vi "MeasuringDevice.Init.vi"(8 "error in (no error)":errorcluster, 11 "LIA.SR810":refnum<class "LIA.SR810.lvclass">) -> (0 "error out":errorcluster, 3 "LIA.SR810 out":refnum<class "LIA.SR810.lvclass">)   [LabVIEW 2017, in "LIA.SR810.lvclass"]
doc: "---------------------------------------------------------------\nJKI State Machine Objects™\nhttp://jki.net/state-machine-objects/\nCopyright (C) 2005-2015, JKI <info@jki.net>\nALL RIGHTS RESERVEDJKI State Machine Objects (SMO) 1.0.0.5\nJKI - JKI\nCopyright (c) 2016, JKI"
uses:
  LIA.SR810.lvclass
  D:/upwork/Laser Measurement Tool/Laser/project/Subsystems/LIA/LIA.lvclass
  Typedefs/Resource--Cluster.ctl
  LIA/LIA.lvclass
  <instrlib>/Stanford Research 830/Stanford Research 830.lvlib
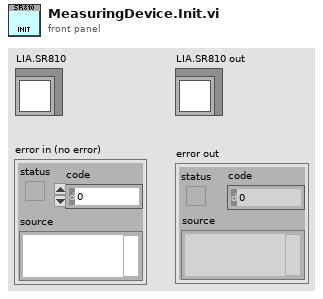
[diagram p1: front panel]
types:
  T1 = typedef "LIA.SR810.lvclass/Resource--Cluster.ctl" = cluster{"VISA resource":refnum<visa-resource-name>}
  T2 = typedef "LIA.lvclass/Configuration--Cluster.ctl" = cluster{"VISA Resource":string}
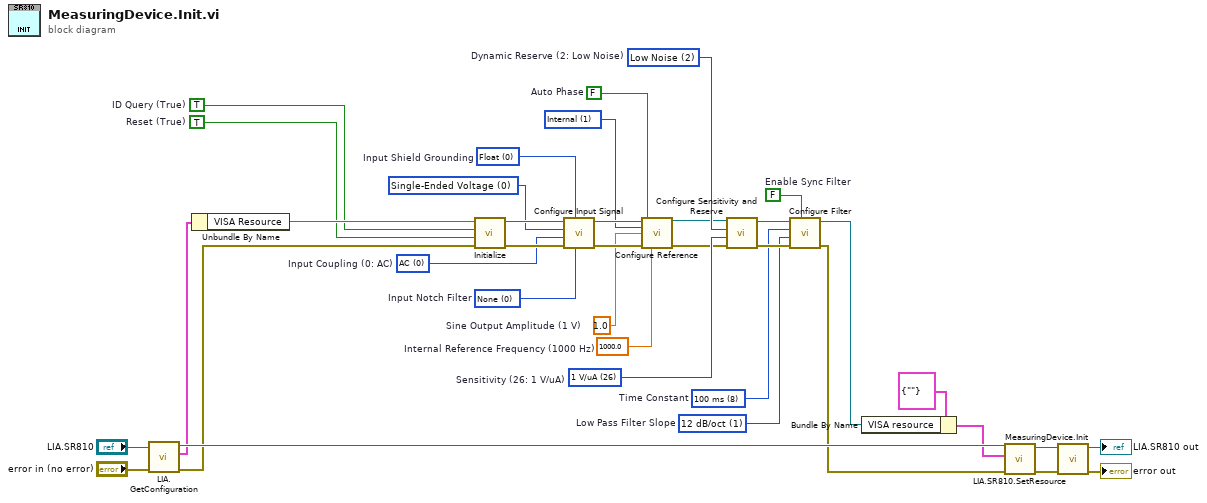
[diagram p0: block diagram]
diagram:
  w1 = TRUE  # Reset (True)
  w2 = TRUE  # ID Query (True)
  w20 = i8 26 items=["Auto Gain"=-1, "2 nV/fA"=0, "5 nV/fA"=1, "10 nV/fA"=2, "20 nV/fA"=3, "50 nV/fA"=4, "100 nV/fA"=5, "200 nV/fA"=6, "500 nV/fA"=7, "1 uV/pA"=8, "2 uV/pA"=9, "5 uV/pA"=10, "10 uV/pA"=11, "20 uV/pA"=12, "50 uV/pA"=13, "100 uV/pA"=14, "200 uV/pA"=15, "500 uV/pA"=16, "1 mV/nA"=17, "2 mV/nA"=18, "5 mV/nA"=19, "10 mV/nA"=20, "20 mV/nA"=21, "50 mV/nA"=22, "100 mV/nA"=23, "200 mV/nA"=24, "500 mV/mA"=25, "1 V/uA"=26]  # Sensitivity (26: 1 V/uA)
  w14 = 1000.0  # Internal Reference Frequency (1000 Hz)
  w15 = 1.0  # Sine Output Amplitude (1 V)
  w24 = u16 0 items=["AC", "DC"]  # Input Coupling (0: AC)
  w25 = u16 0 items=["Single-Ended Voltage", "Differential Voltage", "1 MOhm Current Gain", "100 MOhm Current Gain"] ("Input Connection (0: Single-Ended Voltage)")
  w16 = u16 1 items=["External", "Internal"] ("Reference Source (1: Internal)")
  w19 = i8 2 items=["High Reserve"=0, "Normal"=1, "Low Noise"=2, "Auto Reserve"=-1]  # Dynamic Reserve (2: Low Noise)
  w9 = u16 1 items=["6 dB/oct", "12 dB/oct", "18 db/oct", "24 dB/oct"]  # Low Pass Filter Slope
  w10 = u16 8 items=["10 us", "30 us", "100 us", "300 us", "1 ms", "3 ms", "10 ms", "30 ms", "100 ms", "300 ms", "1 s", "3 s", "10 s", "30 s", "100 s", "300 s", "1 ks", "3 ks", "10 ks", "30 ks"]  # Time Constant
  w11 = FALSE  # Enable Sync Filter
  w21 = FALSE  # Auto Phase
  w22 = u16 0 items=["None", "Line Notch", "2x Line Notch", "Both Notch Filters"]  # Input Notch Filter
  w23 = u16 0 items=["Float", "Ground"]  # Input Shield Grounding
  n1 = call "LIA.GetConfiguration.vi"("error in (no error)"="error in (no error)", "LIA"="LIA.SR810") -> ("error out"=w7:errorcluster, "Configuration"=w30:T2, "LIA out"=w31:refnum<class "LIA.SR810.lvclass">)  [unwired: 7 in]
  n2 = Unbundle By Name(w30) -> ("VISA Resource"=w8:string)
  n3 = call <instrlib>:"Initialize.vi"("error in (no error)"=w7, "Reset (True)"=w1, "ID Query (True)"=w2, "VISA resource name"=w8) -> ("error out"=w29:errorcluster, "VISA resource name out"=w28:refnum<visa-resource-name>)  [unwired: 6 in]
  n4 = call <instrlib>:"Configure Input Signal.vi"("Input Notch Filter (0: None)"=w22, "Input Shield Grounding (0: Float)"=w23, "error in (no error)"=w29, "Input Coupling (0: AC)"=w24, "Input Connection (0: Single-Ended Voltage)"=w25, "VISA resource name"=w28) -> ("error out"=w26:errorcluster, "VISA resource name out"=w27:refnum<visa-resource-name>)  [unwired: 4 in]
  n5 = call <instrlib>:"Configure Reference.vi"("VISA resource name"=w27, "Auto Phase (T: Enabled)"=w21, "Reference Source (1: Internal)"=w16, "Sine Output Amplitude (1 V)"=w15, "error in (no error)"=w26, "Internal Reference Frequency (1000 Hz)"=w14) -> ("VISA resource name out"=w18:refnum<visa-resource-name>, "error out"=w17:errorcluster)  [unwired: 8 in]
  n6 = call <instrlib>:"Configure Sensitivity and Reserve.vi"("error in (no error)"=w17, "Sensitivity (-1: Auto gain)"=w20, "Dynamic Reserve (-1: Auto Reserve)"=w19, "VISA resource name"=w18) -> ("error out"=w13:errorcluster, "VISA resource name out"=w12:refnum<visa-resource-name>)  [unwired: 6 in]
  n7 = call <instrlib>:"Configure Filter.vi"("Enable Sync Filter (F: Disable)"=w11, "error in (no error)"=w13, "Low Pass Filter Slope (1: 12dB/oct)"=w9, "Time Constant (8: 100ms)"=w10, "VISA resource name"=w12) -> ("error out"=w4:errorcluster, "VISA resource name out"=w5:refnum<visa-resource-name>)  [unwired: 5 in]
  n8 = Bundle By Name(cluster=T1 {"VISA resource"=""} ("Resource"), "VISA resource"=w5) -> (w3:T1)
  n9 = call "LIA.SR810.SetResource.vi"("error in (no error)"=w4, "Resource"=w3, "LIA.SR810 in"=w31) -> ("error out"=w33:errorcluster, "LIA.SR810 out"=w32:refnum<class "LIA.SR810.lvclass">)  [unwired: 7 in]
  n10 = call-parent "MeasuringDevice.Init.vi"("error in (no error)"=w33, "MeasuringDevice"=w32) -> ("error out"=→"error out":errorcluster, "MeasuringDevice out"=→"LIA.SR810 out":refnum<class "LIA.SR810.lvclass">)  [unwired: 8 in]
